vi "FC_Test Competition_Team List Builder.vi"   [LabVIEW 2013]
uses:
  <vilib>/Utility/sysdir.llb/System Directory Type.ctl
  FC_Target.ctl
  FC_FIRST Client.lvlib
panel:
  # "This test VI creates an \"FRC Test\" folder on the desktop that it then puts texts file in.\nEach text file will be named with a competition ID# and the data inside the file is ID \nnumbers of all of the teams attending that competition"
types:
  T1 = typedef "FC_FIRST Client.lvlib/FC_Target.ctl" = enum16{"Teams", "Competitions"}
  T2 = typedef "System Directory Type.ctl" = i32
  T3 = enum16{"open", "replace", "create", "open or create", "replace or create", "replace or create with confirmation"}
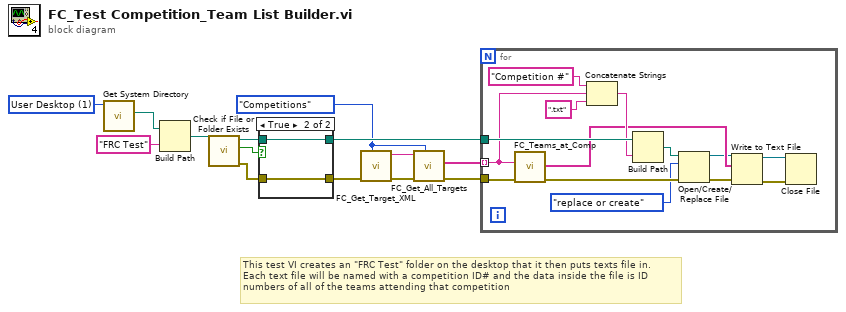
[diagram p0: block diagram]
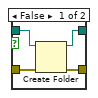
[diagram p2: hidden frame]
diagram:
  w3 = FC_Target."Competitions" ("Target")
  w14 = T2 1 items=["User Home"=0, "User Desktop"=1, "User Documents"=2, "User Application Data"=3, "User Preferences"=4, "User Temporary"=5, "Public Documents"=6, "Public Application Data"=7, "Public Preferences"=8, "Public Cache"=13, "System Core Libraries"=9, "System Installed Libraries"=10, "Application Files"=11, "Boot Volume Root"=12] ("system directory type")
  # "This test VI creates an \"FRC Test\" folder on the desktop that it then puts texts file in.\nEach text file will be named with a competition ID# and the data inside the file is ID \nnumbers of all of the teams attending that competition"
  n1 = call <vilib>:"Get System Directory.vi"("system directory type"=w14) -> ("system directory"=w13:path)  [unwired: 10 in]
  n2 = Build Path(base path=w13, name or relative path="FRC Test") -> (appended path=w11:path)
  n3 = call <vilib>:"Check if File or Folder Exists.vi"("path"=w11) -> ("error out"=w8:errorcluster, "file or folder exists?"=w9:bool, "dup path"=w10:path)  [unwired: 8 in]
  n4 = case shown="True" w9 {
    tunnel: w10 -> [w18 w20]
    tunnel: [w17 w20] -> w7
    tunnel: w8 -> [w16 w19]
    tunnel: [w15 w19] -> w6
    frame False {
      n5 = Create Folder(path (use dialog)=w18, error in=w16) -> (created path=w17:path, error out=w15:errorcluster)  [unwired: 1 in, 1 out]
    }
    frame True {
    }
  }
  n6 = call "FC_Get_Target_XML.vi"("Target"=w3, "error in"=w6) -> ("error out"=w5:errorcluster, "All Teams XML"=w2:string)  [unwired: 8 in]
  n7 = call "FC_Get_All_Targets.vi"("Target"=w3, "Error In"=w5, "Target XML"=w2) -> ("error out"=w4:errorcluster, "Array of Targets"=w1:string[])  [unwired: 6 in, 1 out]
  n8 = for {
    tunnel: w1 -> [w21] mode=indexing
    tunnel: w7 -> [w32]
    tunnel: w4 -> [w34]
    n9 = call "FC_Teams_at_Comp.vi"("error constant"=w34, "Event ID"=w21) -> ("error out"=w29:errorcluster, "Array of Team Numbers"=w26:string[])  [unwired: 8 in]
    n10 = Concatenate Strings("Competition #" ("string"), w21, ".txt" ("string")) -> (w31:string)
    n11 = Build Path(base path=w32, name or relative path=w31) -> (appended path=w30:path)
    n12 = Open/Create/Replace File(file path (use dialog)=w30, error in=w29, operation (0:open)=T3."replace or create") -> (refnum out=w25:refnum<file>, error out=w27:errorcluster)  [unwired: 3 in, 1 out]
    n13 = Write to Text File(file (use dialog)=w25, text=w26, error in=w27) -> (refnum out=w23:refnum<file>, error out=w24:errorcluster)  [unwired: 1 in, 1 out]
    n14 = Close File(refnum=w23, error in=w24) -> ()  [unwired: 2 out]
  }
